vi "Periodic Tasks.vi"(6 "error in":errorcluster, 9 "IR sensor disc":T1) -> ()   [LabVIEW 2012]
doc: "This VI runs in parallel to other tasks. It can contain as many user-defined periodic loops as you need. These can carry out PID or other sorts of timed response."
uses:
  <vilib>/Rock Robotics/SystemInterfaces/AnalogTrigger/FPGA_AnalogTriggerDevRef.ctl
  <vilib>/Rock Robotics/SystemInterfaces/AnalogTrigger/FPGA_AnalogTriggerIndex.ctl
  <vilib>/Rock Robotics/SystemInterfaces/Utilities/FPGA_UtilitiesLED Source.ctl
  <vilib>/Rock Robotics/SystemInterfaces/Utilities/FPGA_UtilitiesLED State.ctl
  Robot Global Data.vi
  <vilib>/Rock Robotics/WPI/Compressor/WPI_CompressorGetSetRefNum.vi
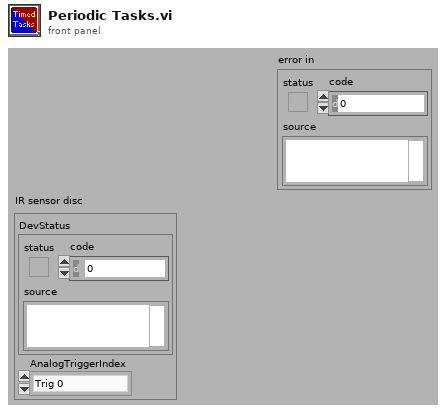
[diagram p1: front panel]
types:
  T1 = typedef "FPGA_AnalogTriggerDevRef.ctl" = cluster{"DevStatus":errorcluster, "AnalogTriggerIndex":T2}
  T2 = typedef "FPGA_AnalogTriggerIndex.ctl" = enum8{"Trig 0", "Trig 1", "Trig 2", "Trig 3", "Trig 4", "Trig 5", "Trig 6", "Trig 7", "Invalid"}
  T3 = typedef "FPGA_UtilitiesLED State.ctl" = enum16{"Off", "On", "Toggle"}
  T4 = typedef "FPGA_UtilitiesLED Source.ctl" = enum16{"User LED", "FPGA LED"}
  T5 = typedef "WPI_CompressorDevRef.ctl" = cluster{"DevStatus":errorcluster, "DigitalInputDevRef":T6, "RelayDevRef":T9}
  T6 = typedef "WPI_DigitalInputDevRef.ctl" = cluster{"DevStatus":errorcluster, "DIO Channel":T7, "Digital Module":T8}
  T7 = typedef "FPGA_DIOChannel.ctl" = enum8{"DIO 1", "DIO 2", "DIO 3", "DIO 4", "DIO 5", "DIO 6", "DIO 7", "DIO 8", "DIO 9", "DIO 10", "DIO 11", "DIO 12", "DIO 13", "DIO 14", "Invalid"}
  T8 = typedef "FPGA_TypedefDigitalModule.ctl" = enum16{"Digital Module 1", "Digital Module 2"}
  T9 = typedef "WPI_RelayDevRef.ctl" = cluster{"DevStatus":errorcluster, "Relay Channel":T10, "Digital Module":T8, "Relay Direction":T11}
  T10 = typedef "FPGA_DIORelayChannel.ctl" = enum8{"Relay 1", "Relay 2", "Relay 3", "Relay 4", "Relay 5", "Relay 6", "Relay 7", "Relay 8", "Invalid"}
  T11 = typedef "WPI_RelayDirection.ctl" = enum16{"Both directions", "Forward only", "Reverse only"}
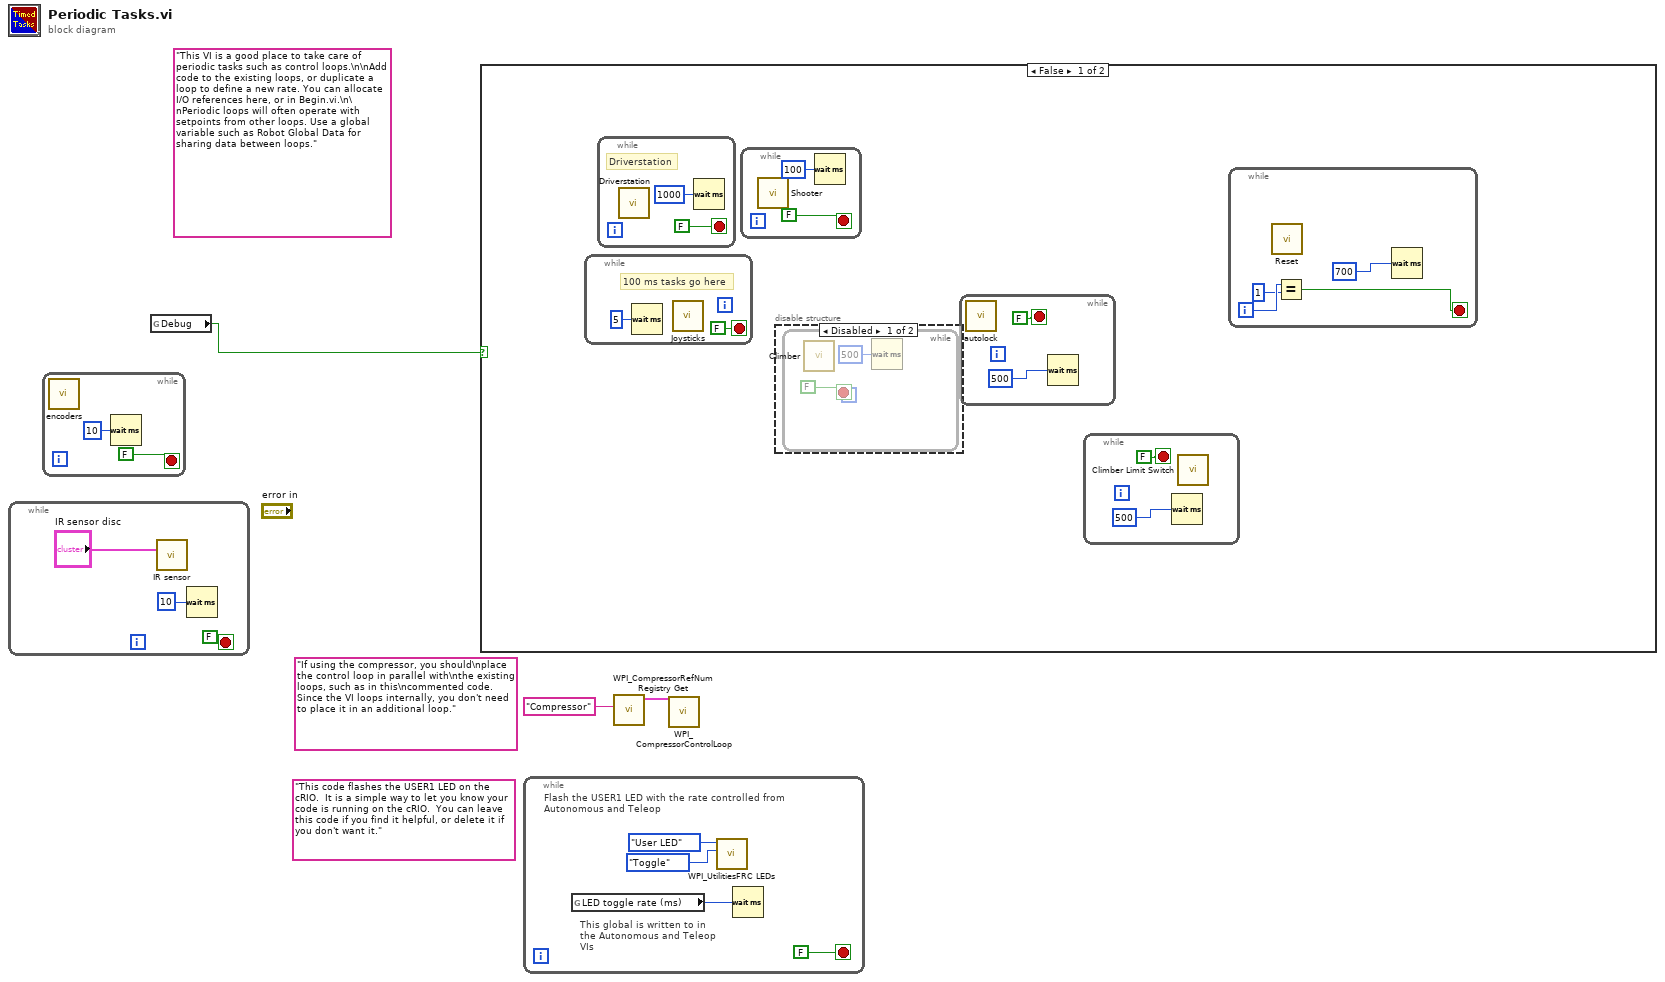
[diagram p0: block diagram]
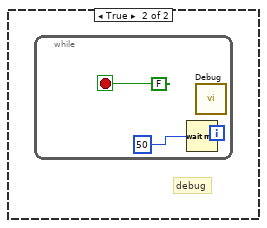
[diagram p3: hidden frame]
diagram:
  (unwired) "If using the compressor, you should\nplace the control loop in parallel with\nthe existing loops, such as in this\ncommented code. Since the VI loops internally, you don't need to place it in an additional loop."
  (unwired) "This code flashes the USER1 LED on the cRIO.  It is a simple way to let you know your code is running on the cRIO.  You can leave this code if you find it helpful, or delete it if you don't want it."
  (unwired) "This VI is a good place to take care of periodic tasks such as control loops.\n\nAdd code to the existing loops, or duplicate a loop to define a new rate. You can allocate I/O references here, or in Begin.vi.\n\nPeriodic loops will often operate with setpoints from other loops. Use a global variable such as Robot Global Data for sharing data between loops."
  n1 = while {
    stop <- FALSE stop-if-true
    n2 = call "IR sensor.vi"("IR sensor disc"="IR sensor disc") -> ()  [unwired: 11 in]
    n3 = Wait (ms)(milliseconds to wait=u32 10) -> ()  [unwired: 1 out]
  }
  n4 = while {
    stop <- FALSE stop-if-true
    n5 = call "encoders.vi"() -> ()  [unwired: 12 in]
    n6 = Wait (ms)(milliseconds to wait=u32 10) -> ()  [unwired: 1 out]
  }
  n7 = global read "Robot Global Data.vi" "Debug"() -> (w1:bool)
  n8 = case shown="False" w1 {
    frame False {
      n9 = while {
        stop <- FALSE stop-if-true
        # "100 ms tasks go here"
        n10 = Wait (ms)(milliseconds to wait=u32 5) -> ()  [unwired: 1 out]
        n11 = call "Joysticks.vi"() -> ()  [unwired: 12 in]
      }
      n12 = while {
        stop <- FALSE stop-if-true
        # "Driverstation"
        n13 = call "Driverstation.vi"() -> ()  [unwired: 12 in]
        n14 = Wait (ms)(milliseconds to wait=u32 1000) -> ()  [unwired: 1 out]
      }
      n15 = while {
        stop <- FALSE stop-if-true
        n16 = call "Shooter.vi"() -> ()  [unwired: 12 in]
        n17 = Wait (ms)(milliseconds to wait=u32 100) -> ()  [unwired: 1 out]
      }
      n18 = disable-structure shown="Disabled" {
        frame Disabled {
          n19 = while {
            stop <- FALSE stop-if-true
            n20 = call "Climber.vi"() -> ()  [unwired: 12 in]
            n21 = Wait (ms)(milliseconds to wait=u32 500) -> ()  [unwired: 1 out]
          }
        }
        frame Enabled {
        }
      }
      n22 = while {
        stop <- FALSE stop-if-true
        n23 = call "autolock.vi"() -> ()  [unwired: 12 in]
        n24 = Wait (ms)(milliseconds to wait=u32 500) -> ()  [unwired: 1 out]
      }
      n25 = while {
        stop <- FALSE stop-if-true
        n26 = Wait (ms)(milliseconds to wait=u32 500) -> ()  [unwired: 1 out]
        n27 = call "Climber Limit Switch.vi"() -> ()  [unwired: 12 in]
      }
      n28 = while {
        i -> [w15]
        stop <- w13 stop-if-true
        n29 = call "Reset.vi"() -> ()  [unwired: 11 in, 1 out]
        n30 = Equal?(x=w15, y=1) -> (x = y?=w13:bool)
        n31 = Wait (ms)(milliseconds to wait=u32 700) -> ()  [unwired: 1 out]
      }
    }
    frame True {
      # "debug"
      n32 = while {
        stop <- FALSE stop-if-true
        n33 = Wait (ms)(milliseconds to wait=u32 50) -> ()  [unwired: 1 out]
        n34 = call "Debug.vi"() -> ()  [unwired: 12 in]
      }
    }
  }
  n35 = while {
    stop <- FALSE stop-if-true
    # "This global is written to in the Autonomous and Teleop VIs"
    # "Flash the USER1 LED with the rate controlled from Autonomous and Teleop"
    n36 = global read "Robot Global Data.vi" "LED toggle rate (ms)"() -> (w27:u32)
    n37 = call <vilib>:"WPI_UtilitiesFRC LEDs.vi"("State"=FPGA_UtilitiesLED_State."Toggle", "LED Type"=FPGA_UtilitiesLED_Source."User LED") -> ()  [unwired: 1 in, 9 out]
    n38 = Wait (ms)(milliseconds to wait=w27) -> ()  [unwired: 1 out]
  }
  n39 = call <vilib>:"WPI_CompressorRefNum Registry Get.vi"("refnum name"="Compressor") -> ("CompressorDevRef"=w3:T5)  [unwired: 9 in, 1 out]
  n40 = call <vilib>:"WPI_CompressorControlLoop.vi"("CompressorDevRef"=w3) -> ()  [unwired: 11 in]
